vi "change_in_sound_speed.vi"(8 "time":dbl format="%#_13g", 9 "Change in Phase":dbl format="%#_13g", 10 "Sample Length":dbl format="%#_13g", 11 "frequency":dbl format="%#_13g") -> (3 "change in speed":dbl format="%#_13g")   [LabVIEW 2016]
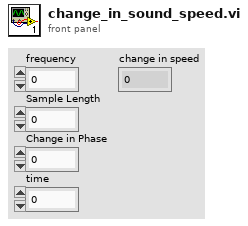
[diagram p1: front panel]
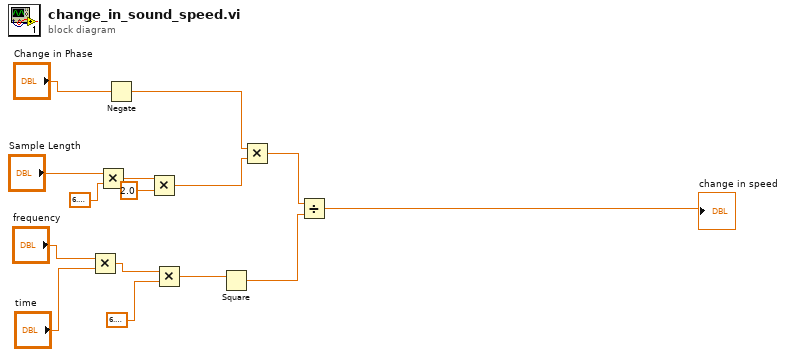
[diagram p0: block diagram]
diagram:
  n1 = Multiply(x="frequency", y="time") -> (x*y=w13:dbl)
  n2 = Multiply(x="Sample Length", y=6.283185307179586) -> (x*y=w9:dbl)
  n3 = Negate(x="Change in Phase") -> (-x=w6:dbl)
  n4 = Multiply(x=w9, y=2.0) -> (x*y=w5:dbl)
  n5 = Multiply(x=w13, y=6.283185307179586) -> (x*y=w3:dbl)
  n6 = Square(x=w3) -> (x^2=w2:dbl)
  n7 = Multiply(x=w6, y=w5) -> (x*y=w4:dbl)
  n8 = Divide(x=w4, y=w2) -> (x/y=→"change in speed":dbl)
